vi "Almost Equal.vi"(0 "X":string, 1 "Condition":string, 5 "error in (no error)":errorcluster, 6 "s":bool, 7 "Unit":string, 8 "Socket":i32, 9 "StepName":string, 10 "timeout ms (-1)":i32=-1, 11 "type":T2, 13 "Station":T1(ring)) -> (19 "error out":errorcluster)   [LabVIEW 2019, in "Unit Test Engine Tools.lvlib"]
uses:
  Unit Test Engine Tools.lvlib
  <vilib>/Utility/Data Type/Type Definitions/Data Type.ctl
  6bbf0a17-1aef-4001-a366-f3d81bf13d00.vi
  LVUT Global 1.vi
  <resource>/objmgr/ni.dex.rc
  <vilib>/Utility/Data Type/NI_Data Type.lvlib
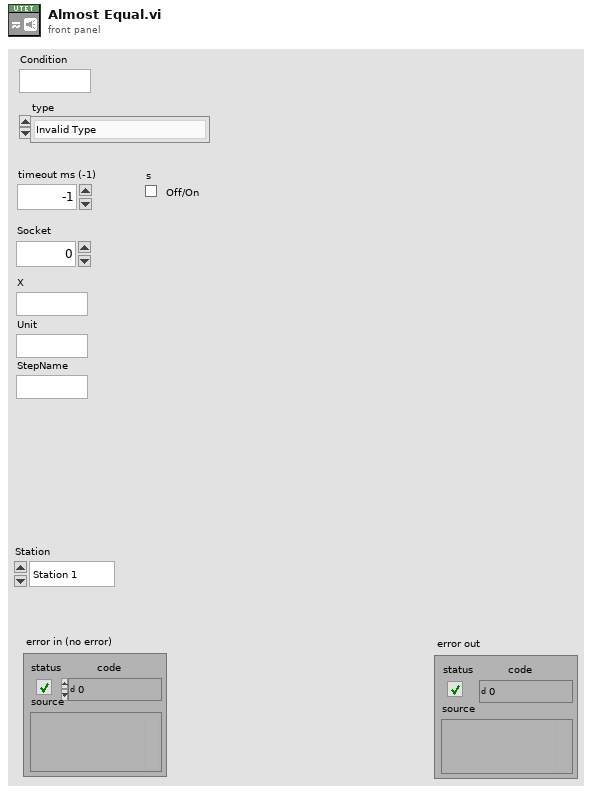
[diagram p1: front panel]
types:
  T1 = enum16{"Station 1", "Station 2", "Station 3", "Station 4"}
  T2 = typedef "NI_Data Type.lvlib/Data Type.ctl" = enum8{"Invalid Type", "Void", "I8", "I16", "I32", "I64", "U8", "U16", "U32", "U64", "Single Float", "Double Float", "Extended Float", "Single Complex", "Double Complex", "Extended Complex", "Enum U8", "Enum U16", "Enum U32", "Enum U64", "Single Float With Unit", "Double Float With Unit", "Extended Float With Unit", "Single Complex with Unit", "Double Complex with Unit", "Extended Complex with Unit", "Boolean", "String", "Path", "Picture", "Tag", "Array", "Cluster", "Variant", "LV Variant", "Waveform", "Timestamp", "Digital Waveform", "Digital Data", "ExpressData", "Refnum", "External Data", "VI", "Poly VI", "LabVIEW Class Instance", "Fixed Point", "Set Collection", "Map Collection"}
  T3 = cluster{"Socket":i32, "Result":string, "Value":string, "Condition":string, "Type":string, "StepName":string, "Error Code":string, "Unit":string}
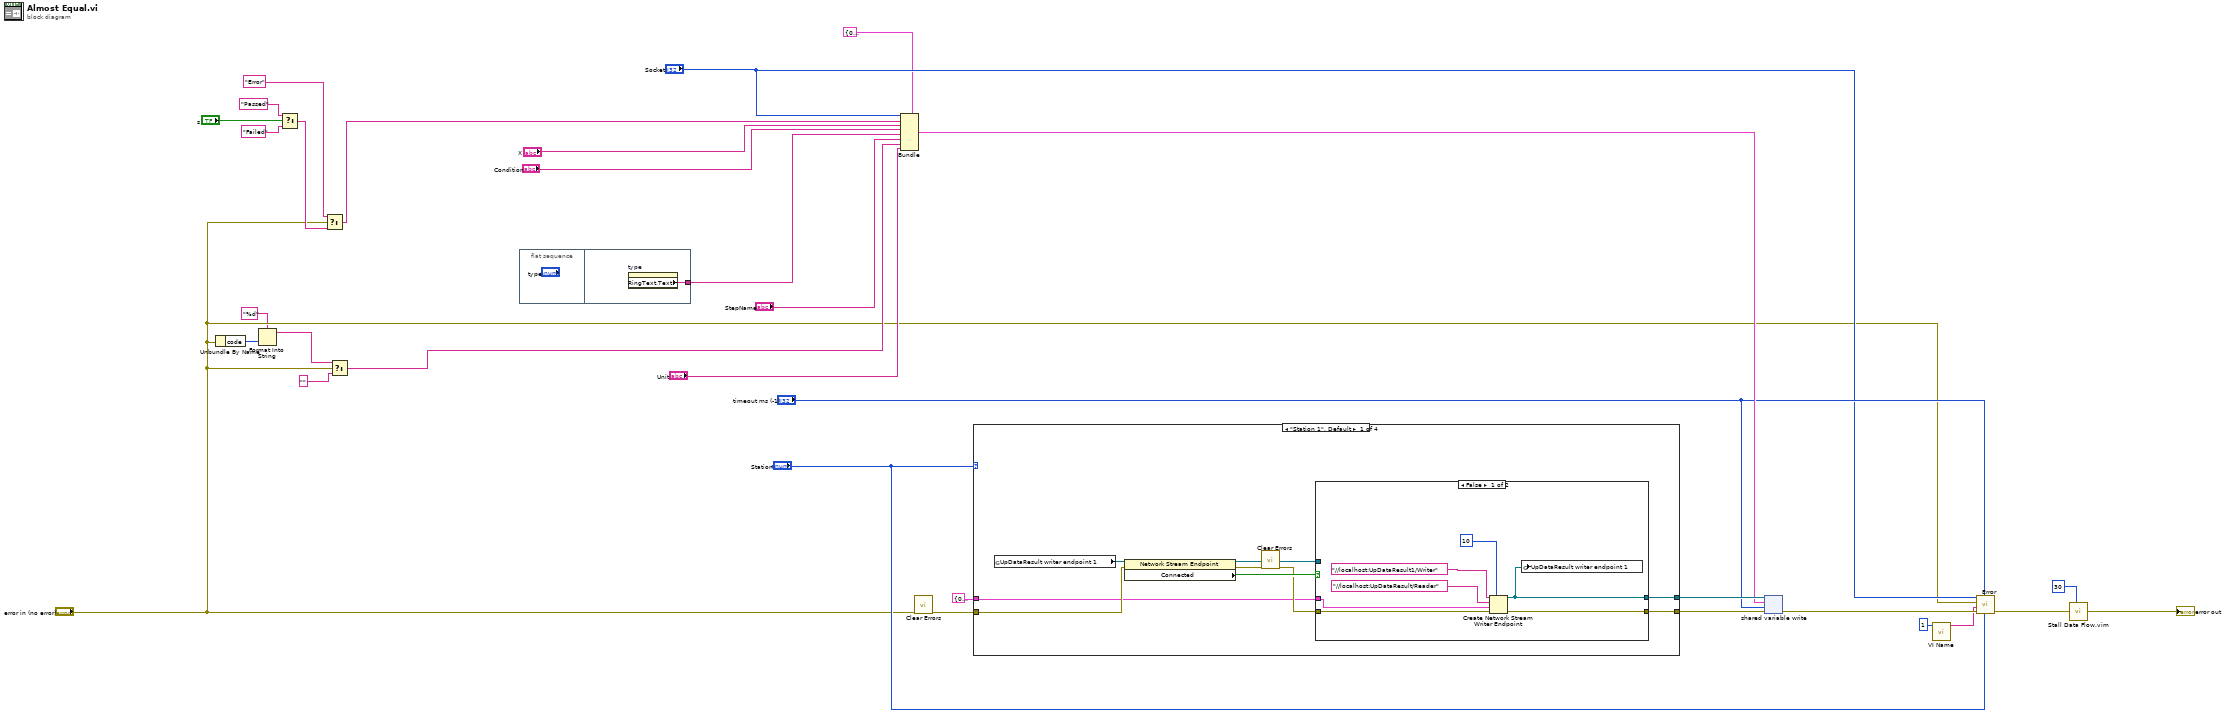
[diagram p0: block diagram]
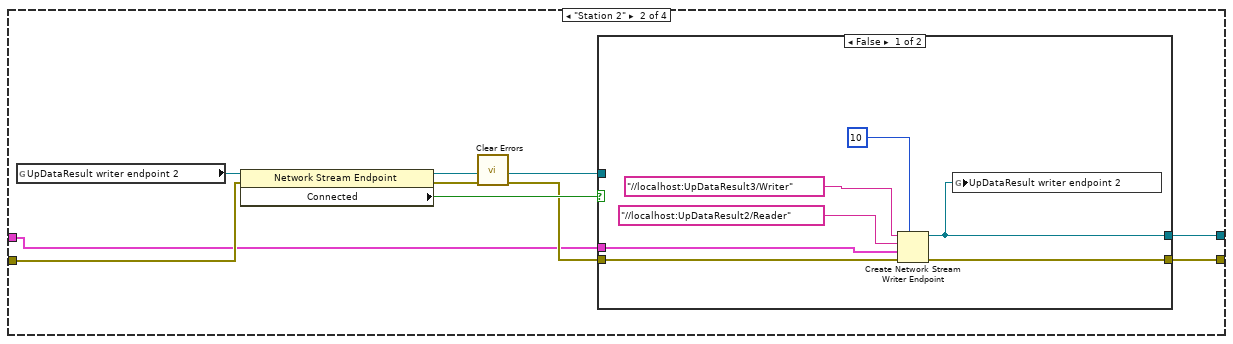
[diagram p3: hidden frame]
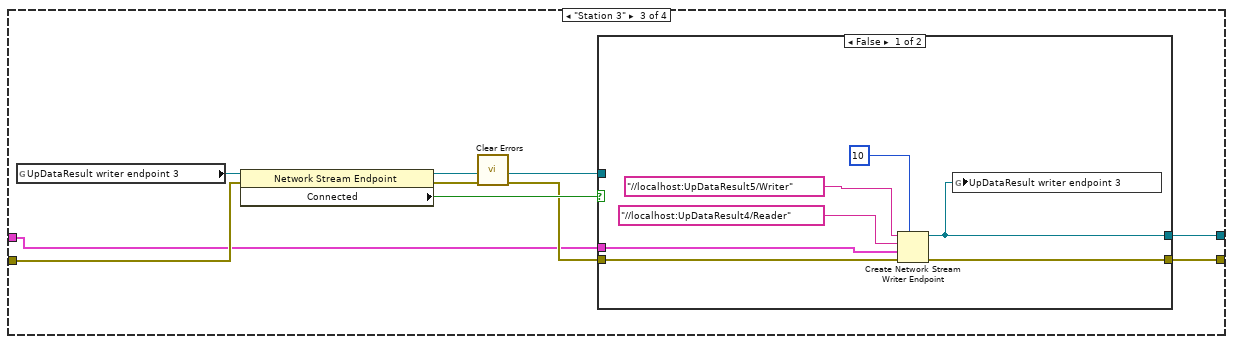
[diagram p5: hidden frame]
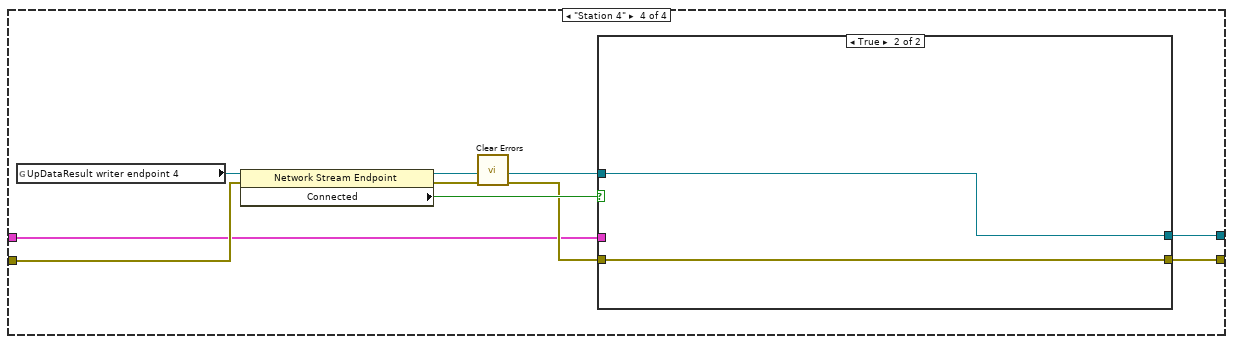
[diagram p7: hidden frame]
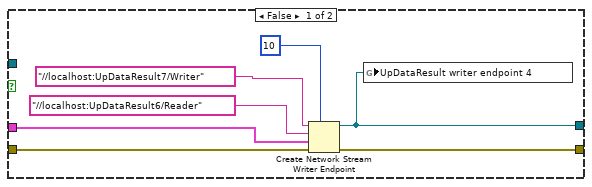
[diagram p8: hidden frame]
diagram:
  n1 = Unbundle By Name("error in (no error)") -> ("code"=w4:i32)
  n2 = Format Into String(format string="%d", w4) -> (resulting string=w2:string)  [unwired: 2 in, 1 out]
  n3 = Select(t="Passed", s="s", f="Failed") -> (s? t:f=w19:string)
  n4 = Select(t="Error", s="error in (no error)", f=w19) -> (s? t:f=w17:string)
  n5 = Select(t=w2, s="error in (no error)", f="") -> (s? t:f=w6:string)
  n6 = flat-sequence {
    tunnel: [w33] -> w24
    frame #0 {
    }
    frame #1 {
      n7 = property on="type" class="Enum (strict)"() -> ("RingText.Text"=w33:string)  [unwired: 2 in, 2 out]
    }
  }
  n8 = Bundle(cluster=T3 {"Socket"=0, "Result"="", "Value"="", "Condition"="", "Type"="", "StepName"="", "Error Code"="", "Unit"=""}, "Socket"="Socket", "Result"=w17, "Value"="X", "Condition"="Condition", "Type"=w24, "StepName"="StepName", "Error Code"=w6, "Unit"="Unit") -> (w21:T3)
  n9 = call <vilib>:"Clear Errors.vi"("error in (no error)"="error in (no error)") -> ("error out"=w20:errorcluster)  [unwired: 5 in, 1 out]
  n10 = case shown="\"Station 1\", Default" "Station" {
    tunnel: [w36 w54 w72 w89] -> w23
    tunnel: w20 -> [w38 w56 w74 w92]
    tunnel: [w35 w53 w71 w90] -> w22
    tunnel: T3 {"Socket"=0, "Result"="", "Value"="", "Condition"="", "Type"="", "StepName"="", "Error Code"="", "Unit"=""} -> [w34 w52 w70 w88]
    frame "Station 1", Default {
      n11 = global read "LVUT Global 1.vi" "UpDataResult writer endpoint 1"() -> (w42:refnum<k21>)
      n12 = property class="Network Stream Endpoint"(reference=w42, error in=w38) -> (reference out=w39:refnum<k21>, error out=w41:errorcluster, "Connected"=w40:bool)
      n13 = call <vilib>:"Clear Errors.vi"("error in (no error)"=w41) -> ("error out"=w37:errorcluster)  [unwired: 5 in, 1 out]
      n14 = case shown="False" w40 {
        tunnel: [w43 w51] -> w35
        tunnel: [w48 w50] -> w36
        tunnel: w37 -> [w45 w50]
        tunnel: w39 -> [_ w51]
        tunnel: w34 -> [w44 _]
        frame False {
          n15 = Create Network Stream Writer Endpoint(7:10 ("writer buffer size"), 8:w45, 9:w44, 10:"//localhost:UpDataResult/Reader" ("reader name"), 11:"//localhost:UpDataResult1/Writer" ("reader name")) -> (0:w48:errorcluster, 3:w43:refnum<k21>)  [unwired: 2 in]
          n16 = global write "LVUT Global 1.vi" "UpDataResult writer endpoint 1"(w43) -> ()
        }
        frame True {
        }
      }
    }
    frame "Station 2" {
      n17 = global read "LVUT Global 1.vi" "UpDataResult writer endpoint 2"() -> (w60:refnum<k21>)
      n18 = property class="Network Stream Endpoint"(reference=w60, error in=w56) -> (reference out=w57:refnum<k21>, error out=w59:errorcluster, "Connected"=w58:bool)
      n19 = call <vilib>:"Clear Errors.vi"("error in (no error)"=w59) -> ("error out"=w55:errorcluster)  [unwired: 5 in, 1 out]
      n20 = case shown="False" w58 {
        tunnel: [w62 w69] -> w53
        tunnel: [w66 w68] -> w54
        tunnel: w55 -> [w63 w68]
        tunnel: w57 -> [_ w69]
        tunnel: w52 -> [w61 _]
        frame False {
          n21 = Create Network Stream Writer Endpoint(7:10 ("writer buffer size"), 8:w63, 9:w61, 10:"//localhost:UpDataResult2/Reader" ("reader name"), 11:"//localhost:UpDataResult3/Writer" ("reader name")) -> (0:w66:errorcluster, 3:w62:refnum<k21>)  [unwired: 2 in]
          n22 = global write "LVUT Global 1.vi" "UpDataResult writer endpoint 2"(w62) -> ()
        }
        frame True {
        }
      }
    }
    frame "Station 3" {
      n23 = global read "LVUT Global 1.vi" "UpDataResult writer endpoint 3"() -> (w78:refnum<k21>)
      n24 = property class="Network Stream Endpoint"(reference=w78, error in=w74) -> (reference out=w75:refnum<k21>, error out=w77:errorcluster, "Connected"=w76:bool)
      n25 = call <vilib>:"Clear Errors.vi"("error in (no error)"=w77) -> ("error out"=w73:errorcluster)  [unwired: 5 in, 1 out]
      n26 = case shown="False" w76 {
        tunnel: [w80 w87] -> w71
        tunnel: [w84 w86] -> w72
        tunnel: w73 -> [w81 w86]
        tunnel: w75 -> [_ w87]
        tunnel: w70 -> [w79 _]
        frame False {
          n27 = Create Network Stream Writer Endpoint(7:10 ("writer buffer size"), 8:w81, 9:w79, 10:"//localhost:UpDataResult4/Reader" ("reader name"), 11:"//localhost:UpDataResult5/Writer" ("reader name")) -> (0:w84:errorcluster, 3:w80:refnum<k21>)  [unwired: 2 in]
          n28 = global write "LVUT Global 1.vi" "UpDataResult writer endpoint 3"(w80) -> ()
        }
        frame True {
        }
      }
    }
    frame "Station 4" {
      n29 = global read "LVUT Global 1.vi" "UpDataResult writer endpoint 4"() -> (w96:refnum<k21>)
      n30 = property class="Network Stream Endpoint"(reference=w96, error in=w92) -> (reference out=w93:refnum<k21>, error out=w95:errorcluster, "Connected"=w94:bool)
      n31 = call <vilib>:"Clear Errors.vi"("error in (no error)"=w95) -> ("error out"=w91:errorcluster)  [unwired: 5 in, 1 out]
      n32 = case shown="True" w94 {
        tunnel: [w98 w105] -> w90
        tunnel: [w102 w104] -> w89
        tunnel: w91 -> [w99 w104]
        tunnel: w93 -> [_ w105]
        tunnel: w88 -> [w97 _]
        frame False {
          n33 = Create Network Stream Writer Endpoint(7:10 ("writer buffer size"), 8:w99, 9:w97, 10:"//localhost:UpDataResult6/Reader" ("reader name"), 11:"//localhost:UpDataResult7/Writer" ("reader name")) -> (0:w102:errorcluster, 3:w98:refnum<k21>)  [unwired: 2 in]
          n34 = global write "LVUT Global 1.vi" "UpDataResult writer endpoint 4"(w98) -> ()
        }
        frame True {
        }
      }
    }
  }
  n35 = shared-variable-write(w22, w23, w21, "timeout ms (-1)") -> (w16:errorcluster)  [unwired: 2 out]
  n36 = call "VI Name.vi"("Level (1)"=1) -> ("VI Name"=w10:string)  [unwired: 9 in, 1 out]
  n37 = call "Error.vi"("Station"="Station", "timeout ms (-1)"="timeout ms (-1)", "error out"=w16, "VI Name"=w10, "error"="error in (no error)", "Socket"="Socket") -> ("error out 2"=w15:errorcluster)  [unwired: 5 in]
  n38 = call "Stall Data Flow.vim"("value in"=w15, "milliseconds to wait"=u32 30) -> ("value out"=→"error out":errorcluster)  [unwired: 1 out]
